vi "Update Series DVR U16.vi"(8 "error in (no error)":errorcluster, 9 "Image #":u32, 10 "image ref array":refnum<data-value>[](array[refnum]), 11 "Series Graph in":refnum<class "Series Graph.lvclass">) -> (0 "error out":errorcluster, 3 "Series Graph out":refnum<class "Series Graph.lvclass">)   [LabVIEW 2023, in "Series Graph.lvclass"]
uses:
  Series Graph.lvclass
  Series Graph.lvclass/Series Graph.ctl
  Detail Graph/Detail Graph.lvclass
  D:/git/Graph-Classes/source/Detail Graph/Detail Graph.lvclass
  D:/git/Graph-Classes/source/Base Graph/Base Graph.lvclass
  D:/git/Graph-Classes/source/Series Graph/Series Graph.lvclass
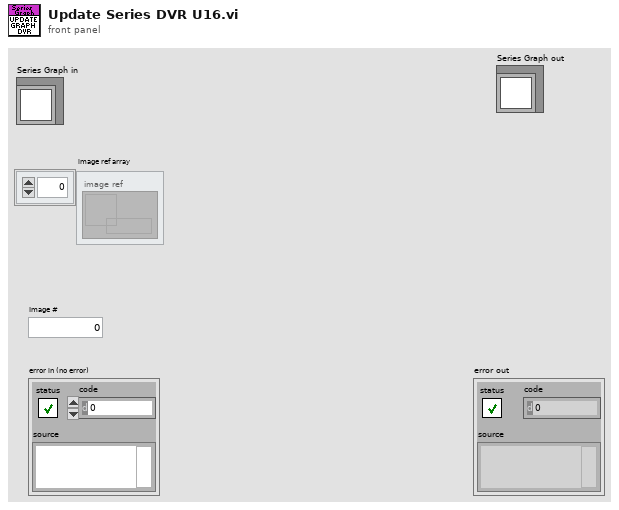
[diagram p1: front panel]
types:
  T1 = typedef "LVPointDoubleTypeDef.ctl" = cluster{"X":dbl, "Y":dbl}
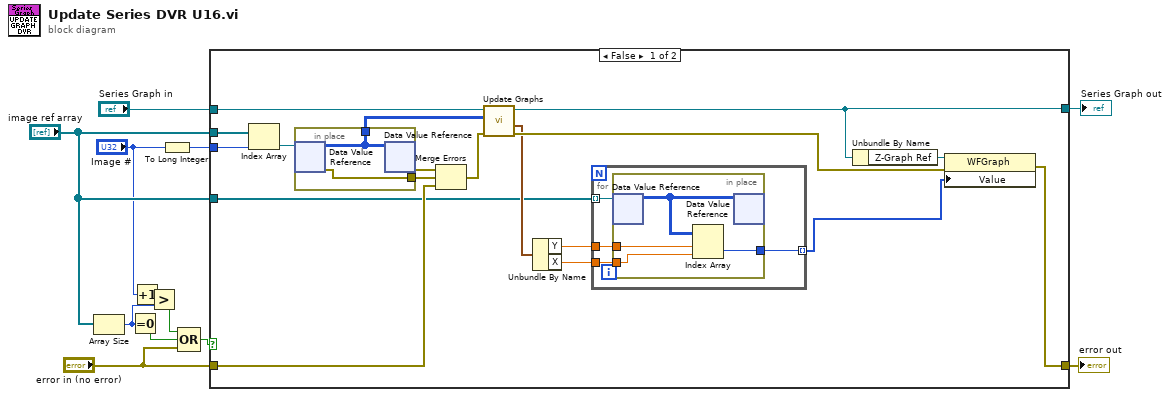
[diagram p0: block diagram]
diagram:
  n1 = Array Size(array="image ref array") -> (size(s)=w2:i32)
  n2 = Equal To 0?(x=w2) -> (x = 0?=w10:bool)
  n3 = Increment(x="Image #") -> (x+1=w1:u32)
  n4 = Greater?(x=w1, y=w2) -> (0:w4:bool)
  n5 = To Long Integer(number="Image #") -> (32bit integer=w6:i32)
  n6 = Compound Arithmetic op=OR(w4, w10, "error in (no error)") -> (w11:bool)
  n7 = case shown="False" w11 {
    tunnel: [w29 w42] -> w12
    tunnel: [w18 w41] -> w7
    tunnel: w6 -> [w26 _]
    tunnel: "error in (no error)" -> [w20 w42]
    tunnel: "Series Graph in" -> [w27 w41]
    tunnel: "image ref array" -> [w25 _]
    tunnel: "image ref array" -> [w16 _]
    frame False {
      n8 = Index Array(array=w25, index=w26) -> (element=w24:refnum<data-value>)
      n9 = in-place {
        in-place-border: [w40] -> w23
        in-place-border: [w39] -> w19
        n10 = in-place-dvr #1(w24) -> (w40:u16[][], w39:errorcluster)
        n11 = in-place-dvr #1(w40) -> (w22:errorcluster)  [unwired: 1 out]
      }
      n12 = Merge Errors(w22, w19, w20) -> (w21:errorcluster)
      n13 = call "Update Graphs.vi"("error in (no error)"=w21, "image"=w23, "Detail Graph in"=w27) -> ("error out"=w30:errorcluster, "Cursor.Cursor Position"=w28:T1, "Detail Graph out"=w18:refnum<class "Series Graph.lvclass">)  [unwired: 6 in]
      n14 = Unbundle By Name(w28) -> ("Y"=w15:dbl, "X"=w14:dbl)
      n15 = for {
        tunnel: w16 -> [w34] mode=indexing
        tunnel: w15 -> [w33]
        tunnel: w14 -> [w32]
        tunnel: [w31] -> w13 mode=indexing
        n16 = in-place {
          in-place-border: w33 -> [w38]
          in-place-border: w32 -> [w37]
          in-place-border: [w36] -> w31
          n17 = in-place-dvr #2(w34) -> (w35:u16[][])  [unwired: 1 out]
          n18 = Index Array(array=w35, index (row)=w38, index (col)=w37) -> (element=w36:u16)
          n19 = in-place-dvr #2(w35) -> ()  [unwired: 2 out]
        }
      }
      n20 = Unbundle By Name(w18) -> ("Z-Graph Ref"=w17:refnum<vi>)
      n21 = property class="WFGraph"(reference=w17, error in=w30, "Value"=w13) -> (error out=w29:errorcluster)  [unwired: 1 out]
    }
    frame True {
    }
  }
  "error out" <- w12
  "Series Graph out" <- w7
